vi "Render.vi"(8 "error in (no error)":errorcluster, 10 "String in":string, 11 "Link in":refnum<class "Link.lvclass">) -> (0 "error out":errorcluster, 2 "String out":string, 3 "Link out":refnum<class "Link.lvclass">)   [LabVIEW 2021, in "Markdown.lvlib" / "Link.lvclass"]
uses:
  Link.lvclass
  C:/GitHub/Markdown/src/Markdown/Markdown.lvclass
  Link.lvclass/Link.ctl
  GetUrl.vi
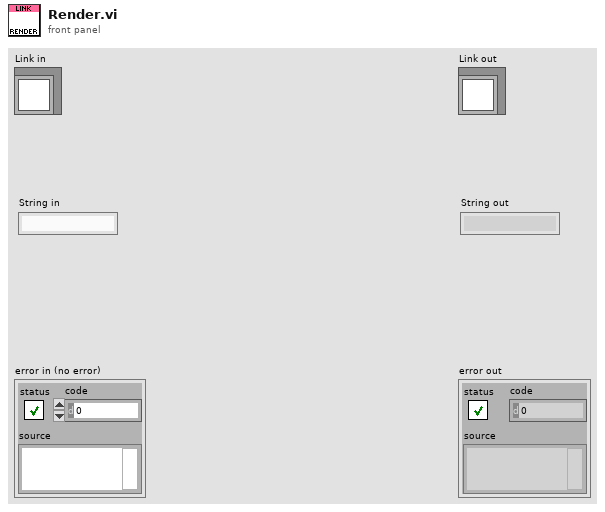
[diagram p1: front panel]
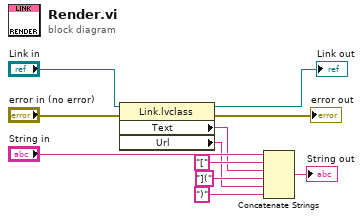
[diagram p0: block diagram]
diagram:
  n1 = property class="Link.lvclass"(reference="Link in", error in="error in (no error)") -> (reference out=→"Link out":refnum<class "Link.lvclass">, error out=→"error out":errorcluster, "Text"=w4:string, "Url"=w2:string)
  n2 = Concatenate Strings("String in", "[" ("string"), w4, "](" ("string"), w2, ")" ("string")) -> (→"String out":string)
